vi "CompareStrings.vi"(10 "Input 2":string, 11 "Input 1":string) -> ()   [LabVIEW 2019, in "StringUtilities.lvlib"]
uses:
  StringUtilities.lvlib
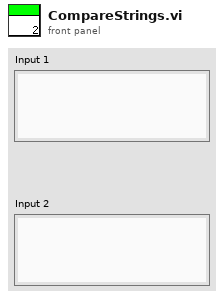
[diagram p1: front panel]
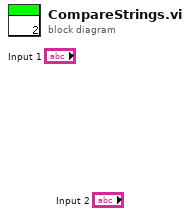
[diagram p0: block diagram]
diagram:
